vi "RefferenceA_Create.vi"(0 "reference in":refnum<class "RefferenceA.lvclass">, 11 "Error In":errorcluster) -> (4 "reference out":refnum<class "RefferenceA.lvclass">, 15 "Error Out":errorcluster)   [LabVIEW 2018, in "RefferenceA.lvclass"]
uses:
  RefferenceA.lvclass
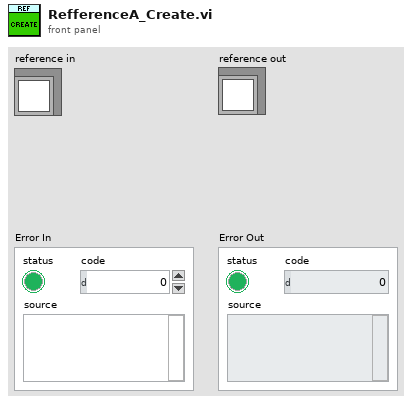
[diagram p1: front panel]
types:
  T1 = typedef "G4BaseTemplate_Simple_5x6x5.lvclass/ObjectAttributes.ctl" = cluster{"Attribute1":dbl}
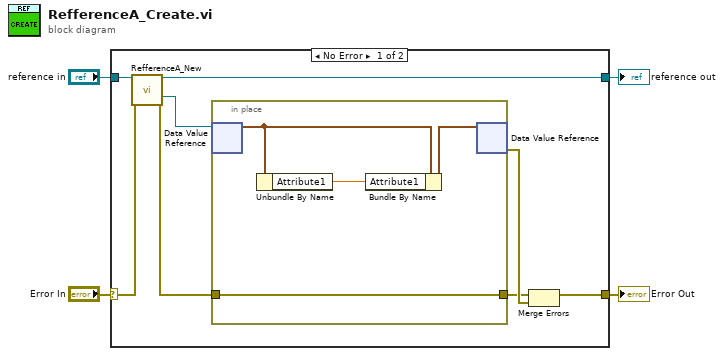
[diagram p0: block diagram]
diagram:
  n1 = case shown="No Error" "Error In" {
    selector: "Error In" -> [w11 w18]
    tunnel: [w5 w18] -> w3
    tunnel: "reference in" -> [w12 w17]
    tunnel: [w10 w17] -> w1
    frame No Error {
      n2 = call "RefferenceA_New.vi"("reference in"=w12, "error in (no error)"=w11) -> ("reference out"=w10:refnum<class "RefferenceA.lvclass">, "DVRRefOut"=w8:refnum<data-value>, "error out"=w7:errorcluster)  [unwired: 10 in, 1 out]
      n3 = in-place {
        in-place-border: w7 -> [w13]
        in-place-border: [w13] -> w6
        n4 = in-place-dvr #1(w8) -> (w15:T1)  [unwired: 1 out]
        n5 = Unbundle By Name(w15) -> ("Attribute1"=w14:dbl)
        n6 = Bundle By Name(cluster=w15, "Attribute1"=w14) -> (w16:T1)
        n7 = in-place-dvr #1(w16) -> (w9:errorcluster)  [unwired: 1 out]
      }
      n8 = Merge Errors(w6, w9) -> (w5:errorcluster)
    }
    frame Error {
      # "VI-TechBaseTemplate_Simple_4x4x4"
    }
  }
  "Error Out" <- w3
  "reference out" <- w1
